vi "Create.vi"(10 "Value":variant) -> (3 "Variant out":refnum<class "Variant.lvclass">)   [LabVIEW 2020, in "Promises.lvlib" / "Variant.lvclass"]
uses:
  Variant.lvclass
  Variant.lvclass/Variant.ctl
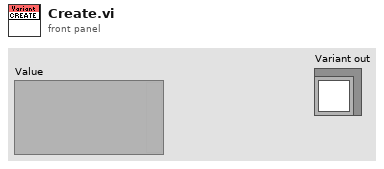
[diagram p1: front panel]
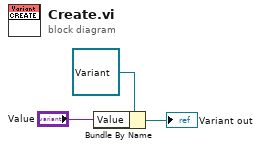
[diagram p0: block diagram]
diagram:
  n1 = Bundle By Name(cluster=refnum<class "Variant.lvclass"> refnum ("Variant in"), "Value"="Value") -> (→"Variant out":refnum<class "Variant.lvclass">)
